vi "Is Locked.vi"(8 "error in (no error)":errorcluster, 11 "SQLite in":refnum<class "SQLite.lvclass">) -> (0 "error out":errorcluster, 2 "Is Locked?":bool, 3 "SQLite out":refnum<class "SQLite.lvclass">)   [LabVIEW 2020, in "Summer of LabVIEW.lvlib" / "SQLite.lvclass"]
uses:
  SQLite.lvclass
  SQLite.lvclass/SQLite.ctl
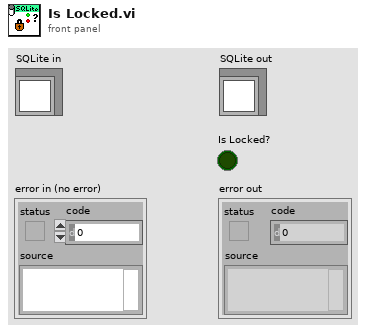
[diagram p1: front panel]
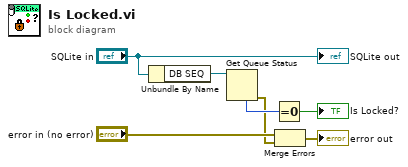
[diagram p0: block diagram]
diagram:
  n1 = Unbundle By Name("SQLite in") -> ("DB SEQ"=w5:refnum<queue>)
  n2 = Get Queue Status(queue=w5) -> (error out=w1:errorcluster, # elements in queue=w4:i32)  [unwired: 2 in, 6 out]
  n3 = Equal To 0?(x=w4) -> (x = 0?=→"Is Locked?":bool)
  n4 = Merge Errors("error in (no error)", w1) -> (→"error out":errorcluster)
  "SQLite out" <- "SQLite in"
